vi "queue test server.vi"() -> ()   [LabVIEW 2021]
panel:
  out "error out":errorcluster
  out "element":dbl[][](array[numeric])
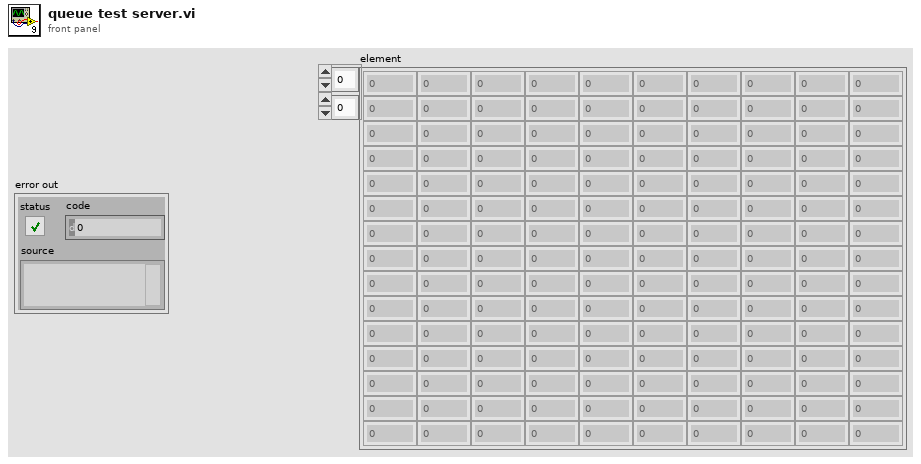
[diagram p1: front panel]
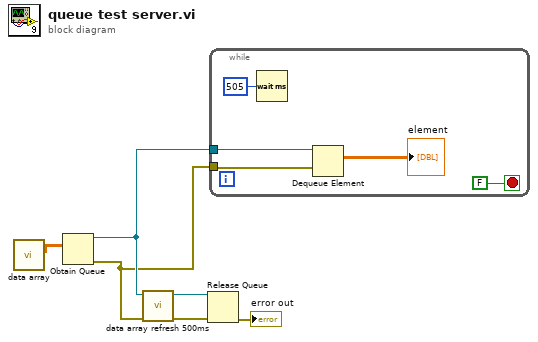
[diagram p0: block diagram]
diagram:
  n1 = call "data array.vi"() -> ("Array"=w6:dbl[][])  [unwired: 11 in]
  n2 = Obtain Queue(element data type=w6) -> (queue out=w5:refnum<queue>, error out=w1:errorcluster)  [unwired: 4 in, 1 out]
  n3 = call "data array refresh 500ms.vi"("error in (no error)"=w1, "queue out"=w5) -> ("error out"=w3:errorcluster, "queue out 2"=w4:refnum<queue>)  [unwired: 8 in]
  n4 = Release Queue(queue=w4, error in (no error)=w3) -> (error out=→"error out":errorcluster)  [unwired: 1 in, 2 out]
  n5 = while {
    tunnel: w5 -> [w10]
    tunnel: w1 -> [w9]
    stop <- FALSE stop-if-true
    n6 = Wait (ms)(milliseconds to wait=u32 505) -> ()  [unwired: 1 out]
    n7 = Dequeue Element(queue=w10, error in (no error)=w9) -> (element=→"element":dbl[][])  [unwired: 1 in, 3 out]
  }
